vi "Open Command (Core).vi"(0 "SLSC Remote in":refnum<class "SLSC Remote.lvclass">, 5 "resource":string, 7 "command in":refnum<k21>, 11 "error in (no error)":errorcluster) -> (4 "SLSC Remote out":refnum<class "SLSC Remote.lvclass">, 8 "command out":refnum<k21>, 15 "error out":errorcluster)   [LabVIEW 2015, in "SLSC Remote.lvclass"]
uses:
  SLSC Remote.lvclass
  <vilib>/NI/i3 JSON/JSON Generation/Create Value Files/Create Value - Object.vi
  <vilib>/NI/i3 JSON/JSON Generation/Add Object Parameter Files/Add Object Parameter - String.vi
  <vilib>/NI/NI JSONRPC Server Framework/Classes/Server/Format Client Request (Auto-Increment).vi
  <vilib>/httpClient/POSTBuffer.vi
  <vilib>/NI/NI JSONRPC Server Framework/Classes/Server/JSONRPC Server.lvclass
  <vilib>/NI/i3 JSON/i3-json.lvlib
  <vilib>/httpClient/LabVIEWHTTPClient.lvlib
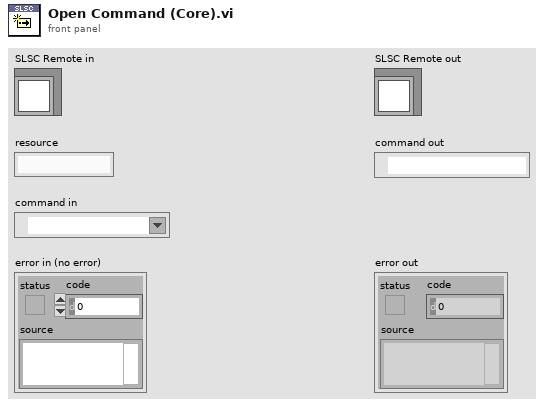
[diagram p1: front panel]
types:
  T1 = typedef "LabVIEWHTTPClient.lvlib/ClientHandle.ctl" = refnum<k1>
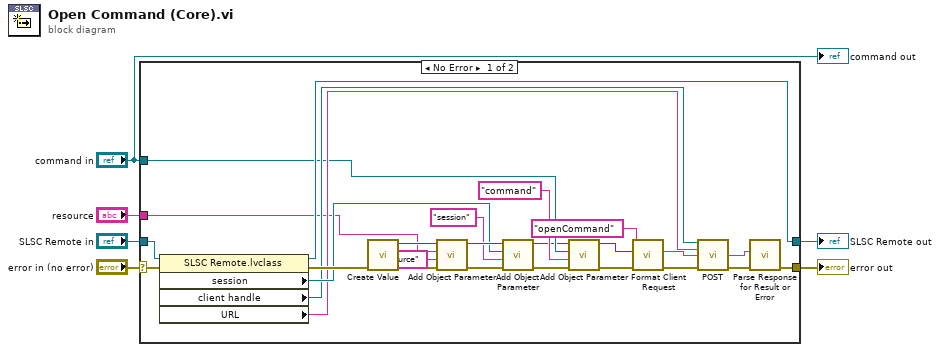
[diagram p0: block diagram]
diagram:
  n1 = case shown="No Error" "error in (no error)" {
    selector: "error in (no error)" -> [w29 w33]
    tunnel: "command in" -> [w13 _]
    tunnel: "SLSC Remote in" -> [w31 w34]
    tunnel: [w30 w34] -> w3
    tunnel: [w16 w33] -> w1
    tunnel: "resource" -> [w15 _]
    frame No Error {
      n2 = property class="SLSC Remote.lvclass"(reference=w31, error in=w29) -> (reference out=w30:refnum<class "SLSC Remote.lvclass">, error out=w28:errorcluster, "session"=w23:refnum<k21>, "client handle"=w21:T1, "URL"=w20:string)
      n3 = call-poly <vilib>:"Create Value.vi"("error in (no error)"=w28) -> ("error out"=w27:errorcluster, "JSON Tree"=w32:variant)  [unwired: 9 in]
      n4 = call-poly <vilib>:"Add Object Parameter.vi"("error in (no error)"=w27, "Name"="resource", "String"=w15, "JSON Tree in (JSON Object)"=w32) -> ("error out"=w26:errorcluster, "JSON Tree out (JSON Object)"=w24:variant)  [unwired: 6 in]
      n5 = call-poly <vilib>:"Add Object Parameter.vi"("error in (no error)"=w26, "Name"="session", "String"=w23, "JSON Tree in (JSON Object)"=w24) -> ("error out"=w11:errorcluster, "JSON Tree out (JSON Object)"=w12:variant)  [unwired: 6 in]
      n6 = call-poly <vilib>:"Add Object Parameter.vi"("error in (no error)"=w11, "Name"="command", "String"=w13, "JSON Tree in (JSON Object)"=w12) -> ("error out"=w9:errorcluster, "JSON Tree out (JSON Object)"=w10:variant)  [unwired: 6 in]
      n7 = call-poly <vilib>:"Format Client Request.vi"("error in (no error)"=w9, "params"=w10, "method"="openCommand") -> ("error out"=w19:errorcluster, "Request String"=w25:string)  [unwired: 7 in]
      n8 = call-poly <vilib>:"POST.vi"("client handle"=w21, "url"=w20, "buffer"=w25, "error in (no error)"=w19) -> ("body"=w18:string, "error out"=w17:errorcluster)  [unwired: 8 in, 2 out]
      n9 = call <vilib>:"Parse Response for Result or Error.vi"("error in"=w17, "Response String In"=w18) -> ("error out"=w16:errorcluster)  [unwired: 8 in, 1 out]
    }
    frame Error {
    }
  }
  "error out" <- w1
  "SLSC Remote out" <- w3
  "command out" <- "command in"
